vi "MGI Bezier Weights (DBL).vi"(1 "u":dbl format="%.2f") -> (0 "Bezier Weights":dbl[](array[numeric]) format="%.2f")   [LabVIEW 2016]
doc: "Computes an array of four weights, (1-u)^3, 3u(1-u)^2, 3u^2(1-u), and u^3 given u. u should be between 0 and 1.\n\nAuthored by David A. Moore\nsupport@mooregoodideas.com\nwww.mooregoodideas.com\n\nCopyright (c) 2010, Moore Good Ideas, Inc.\n\nAll rights reserved.\n\nRedistribution and use in source and binary forms, with or without modification, are permitted provided that the following conditions are met:\n\n * Redistributions of source code must retain the above copyright notice, this list of conditions and the following disclaimer.\n * Redistributions in binary form must reproduce the above copyright notice, this list of conditions and the following disclaimer in the documentation and/or other materials provided with the distribution.\n * Neither the name of Moore Good Ideas, Inc. nor the names of its contributors may be used to endorse or promote products derived from this software without specific prior written permission.\n\nTHIS SOFTWARE IS PROVIDED BY THE COPYRIGHT HOLDERS AND CONTRIBUTORS \"AS IS\" AND ANY EXPRESS OR IMPLIED WARRANTIES, INCLUDING, BUT NOT LIMITED TO, THE IMPLIED WARRANTIES OF MERCHANTABILITY AND FITNESS FOR A PARTICULAR PURPOSE ARE DISCLAIMED. IN NO EVENT SHALL THE COPYRIGHT OWNER OR CONTRIBUTORS BE LIABLE FOR ANY DIRECT, INDIRECT, INCIDENTAL, SPECIAL, EXEMPLARY, OR CONSEQUENTIAL DAMAGES (INCLUDING, BUT NOT LIMITED TO, PROCUREMENT OF SUBSTITUTE GOODS OR SERVICES; LOSS OF USE, DATA, OR PROFITS; OR BUSINESS INTERRUPTION) HOWEVER CAUSED AND ON ANY THEORY OF LIABILITY, WHETHER IN CONTRACT, STRICT LIABILITY, OR TORT (INCLUDING NEGLIGENCE OR OTHERWISE) ARISING IN ANY WAY OUT OF THE USE OF THIS SOFTWARE, EVEN IF ADVISED OF THE POSSIBILITY OF SUCH DAMAGE."
panel:
  # "(1-u)^3"
  # "3u*(1-u)^2"
  # "3u^2*(1-u)"
  # "u^3"
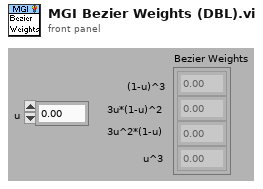
[diagram p1: front panel]
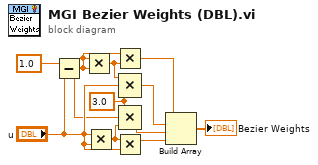
[diagram p0: block diagram]
diagram:
  w2 = 3.0 ("Input")
  n1 = Subtract(x=1.0, y="u") -> (x-y=w5:dbl)
  n2 = Multiply(x=w5, y=w5) -> (x*y=w8:dbl)
  n3 = Multiply(x="u", y="u") -> (x*y=w6:dbl)
  n4 = Multiply(x=w5, y=w8) -> (x*y=w9:dbl)
  n5 = Multiply(x=w6, y="u") -> (x*y=w11:dbl)
  n6 = Compound Arithmetic op=MULTIPLY(w8, "u", w2) -> (w3:dbl)
  n7 = Compound Arithmetic op=MULTIPLY(w2, w5, w6) -> (w4:dbl)
  n8 = Build Array(w9, w3, w4, w11) -> (→"Bezier Weights":dbl[])
